vi "GetTabControls.vi"(7 "controls":i32[](array[numeric]), 9 "PythonConverter_GUI in":refnum<class "PythonConverter_GUI.lvclass">) -> (3 "PythonConverter_GUI out":refnum<class "PythonConverter_GUI.lvclass">, 4 "classes":string[](array[string]), 5 "create_controls":string)   [LabVIEW 2014, in "Raspberry Pi Compatible Compiler for LabVIEW.lvlib" / "PythonConverter_GUI.lvclass"]
uses:
  PythonConverter_GUI.lvclass
  Parsing/ClassTypeTD.ctl
  PythonConverter_GUI.lvclass/PythonConverter_GUI.ctl
  VI Interpreter/Classes/Control/Control.lvclass
  VI Interpreter/Classes/VI Interpreter/VI Interpreter.lvclass
  Parsing/Python Functions.lvlib
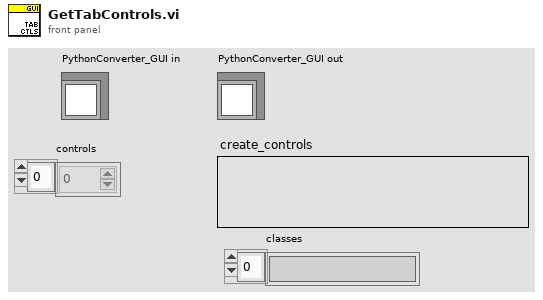
[diagram p1: front panel]
types:
  T1 = typedef "Raspberry Pi Compatible Compiler for LabVIEW.lvlib/Python Functions.lvlib/ClassTypeTD.ctl" = enum16{"class", "function"}
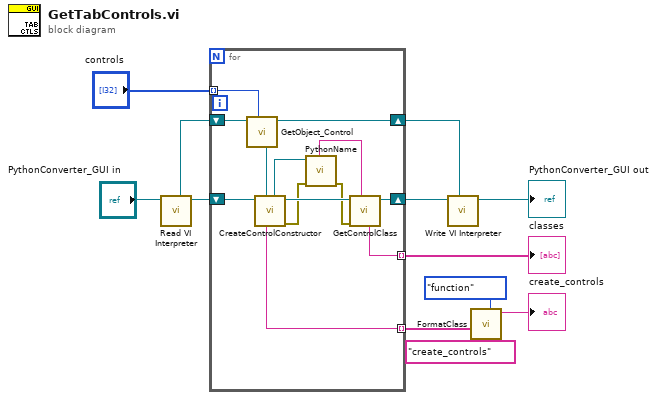
[diagram p0: block diagram]
diagram:
  n1 = call "Read VI Interpreter.vi"("PythonConverter_GUI in"="PythonConverter_GUI in") -> ("PythonConverter_GUI out"=w4:refnum<class "PythonConverter_GUI.lvclass">, "VI Interpreter"=w3:refnum<class "VI Interpreter.lvclass">)  [unwired: 7 in]
  n2 = for {
    tunnel: "controls" -> [w24] mode=indexing
    shift-right: [w19] -> w7
    shift-left: w3 -> [w25]
    shift-right: [w23] -> w8
    shift-left: w4 -> [w18]
    tunnel: [w21] -> w1 mode=indexing
    tunnel: [w20] -> w2 mode=indexing
    n3 = call "GetObject_Control.vi"("UID"=w24, "VI Interpreter in"=w25) -> ("VI Interpreter out"=w19:refnum<class "VI Interpreter.lvclass">, "control"=w16:refnum<class "Control.lvclass">)  [unwired: 4 in, 2 out]
    n4 = call "CreateControlConstructor.vi"("Control in"=w16, "PythonConverter_GUI in"=w18) -> ("error out"=w14:errorcluster, "PythonConverter_GUI out"=w17:refnum<class "PythonConverter_GUI.lvclass">, "Control out"=w13:refnum<class "Control.lvclass">, "control"=w20:string)  [unwired: 5 in, 1 out]
    n5 = call-dynamic "PythonName.vi"("error in"=w14, "GObject in"=w13) -> ("error out"=w15:errorcluster, "UID"=w22:string)  [unwired: 6 in, 2 out]
    n6 = call "GetControlClass.vi"("name"=w22, "error in"=w15, "PythonConverter_GUI in"=w17) -> ("PythonConverter_GUI out"=w23:refnum<class "PythonConverter_GUI.lvclass">, "class"=w21:string)  [unwired: 4 in, 1 out]
  }
  "classes" <- w1
  n7 = call "Write VI Interpreter.vi"("VI Interpreter"=w7, "PythonConverter_GUI in"=w8) -> ("PythonConverter_GUI out"=→"PythonConverter_GUI out":refnum<class "PythonConverter_GUI.lvclass">)  [unwired: 7 in]
  n8 = call "FormatClass.vi"("type"=ClassTypeTD."function", "name"="create_controls", "body"=w2) -> ("python"=→"create_controls":string)  [unwired: 8 in]
